vi "get_storage_mode.vi"(8 "error in (no error)":errorcluster, 11 "Image.lvclass in":refnum<class "Image.lvclass">) -> (0 "error out":errorcluster, 2 "storage mode":T1, 3 "Image.lvclass out":refnum<class "Image.lvclass">)   [LabVIEW 2010, in "Image.lvclass"]
uses:
  Image.lvclass
  storage_mode.ctl
  Image.lvclass/Image.ctl
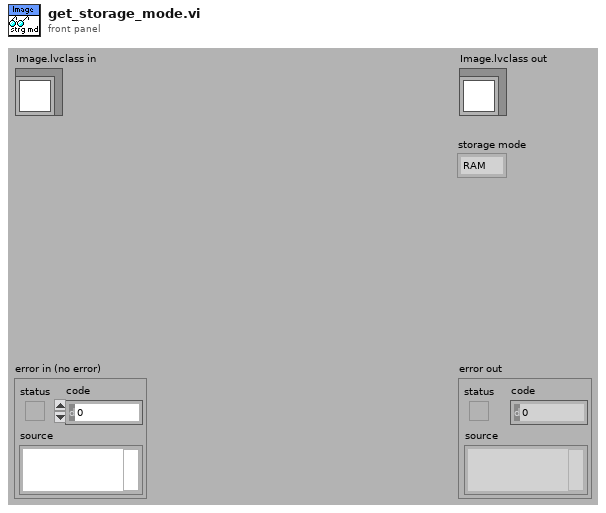
[diagram p1: front panel]
types:
  T1 = typedef "Image.lvclass/storage_mode.ctl" = enum16{"RAM", "disk"}
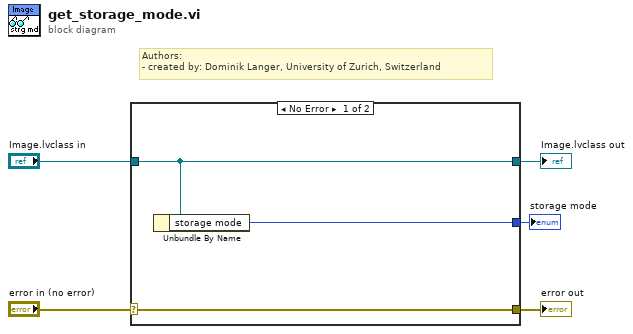
[diagram p0: block diagram]
diagram:
  # "Authors: \n- created by: Dominik Langer, University of Zurich, Switzerland"
  n1 = case shown="No Error" "error in (no error)" {
    selector: "error in (no error)" -> [w8 w9]
    tunnel: [w8 w9] -> w4
    tunnel: [w7 w10] -> w2
    tunnel: "Image.lvclass in" -> [w7 w10]
    tunnel: [w6 _] -> w1
    frame No Error {
      n2 = Unbundle By Name(w7) -> ("storage mode"=w6:T1)
    }
    frame Error {
    }
  }
  "error out" <- w4
  "Image.lvclass out" <- w2
  "storage mode" <- w1
